vi "Get Slot.vi"(8 "error in":errorcluster, 11 "slot ref in":T1 format="%.0x") -> (0 "error out":errorcluster, 2 "module":refnum<class "Module.lvclass">, 3 "slot ref out":T1 format="%.0x")   [LabVIEW 2017, in "Scan Engine Scripting.lvlib"]
uses:
  Scan Engine Scripting.lvlib
  <vilib>/NI Veristand/Custom Device API/Custom Device Item Ref.ctl
  Modules.lvlibp/niveristand-scan-engine-ethercat-custom-device/Custom Device Source/Scripting/Modules/Module/Module.lvclass
  Modules.lvlibp/niveristand-scan-engine-module-libraries/Source/RSI Module/RSI Module.lvclass
  <vilib>/NI Veristand/Custom Device API/Custom Device API.lvlib
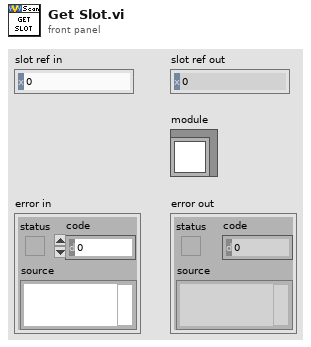
[diagram p1: front panel]
types:
  T1 = typedef "Custom Device API.lvlib/Custom Device Item Ref.ctl" = u64
  T2 = typedef "Modules.lvlibp/Custom Device API.lvlib/Custom Device Item Ref.ctl" = u64
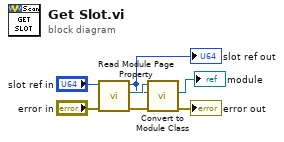
[diagram p0: block diagram]
diagram:
  n1 = call "Read Module Page Property.vi"("error in (no error)"="error in", "Node Ptr In"="slot ref in") -> ("error out"=w3:errorcluster, "RSI Module"=w5:refnum<class "RSI Module.lvclass">, "Node Ptr Out"=w4:T2)  [unwired: 7 in]
  "slot ref out" <- w4
  n2 = call-dynamic "Convert to Module Class.vi"("error in"=w3, "slot ref in"=w4, "RSI Module in"=w5) -> ("error out"=→"error out":errorcluster, "module"=→"module":refnum<class "Module.lvclass">)  [unwired: 6 in, 1 out]
